vi "Write Parent Attributes.vi"(10 "Parent Attributes":refnum<data-value>, 11 "Actor in":refnum<class "Actor.lvclass">) -> (3 "Actor out":refnum<class "Actor.lvclass">)   [LabVIEW 2020, in "jettl.lvlib" / "Actor.lvclass"]
uses:
  Actor.lvclass
  Msg/Msg.lvclass
  Transport/Transport.lvclass
  Actor Attributes.ctl
  jettl.lvlib
  Msgs.ctl
  Msg Names.ctl
  Unified Layer.ctl
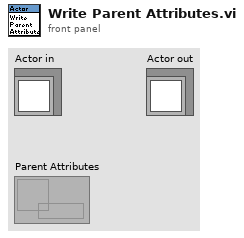
[diagram p1: front panel]
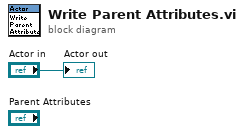
[diagram p0: block diagram]
diagram:
  "Actor out" <- "Actor in"
